vi "LVClass info.vi"(8 "error in (no error)":errorcluster, 11 "Variant":variant) -> (0 "error out":errorcluster, 3 "child strings":string[](array[string]))   [LabVIEW 2017, in "Variant Tree API.lvlib"]
uses:
  Variant Tree/Source/Variant Tree API.lvlib
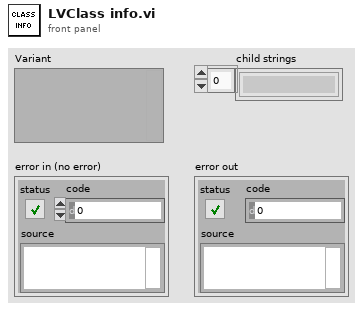
[diagram p1: front panel]
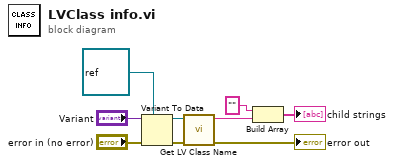
[diagram p0: block diagram]
diagram:
  n1 = Variant To Data(error in="error in (no error)", type=refnum<class> refnum ("LabVIEW Object"), Variant="Variant") -> (data=w7:refnum<class>, error out=w3:errorcluster)
  n2 = call <vilib>:"Get LV Class Name.vi"("error in (no error)"=w3, "object"=w7) -> ("error out"=→"error out":errorcluster, "class name"=w8:string)  [unwired: 8 in]
  n3 = Build Array("" ("element"), w8) -> (→"child strings":string[])
